vi "test4.vi"() -> ()   [LabVIEW 2014]
uses:
  <vilib>/sound2/lvsound2.llb/Sound Data Format.ctl
  <vilib>/sound2/lvsound2.llb/Sound Output Set Volume (Single).vi
  <vilib>/Utility/inputDevices.llb/keyboardAcquire.vi
  <vilib>/sound2/lvsound2.llb/Sound Output Write (DBL Single).vi
  <vilib>/Utility/inputDevices.llb/closeKeyboard.vi
  <vilib>/measure/NI_MABase.lvlib
panel:
  out "element":T1(ring)
  in  "volume":dbl=100.0
  in  "stop":bool
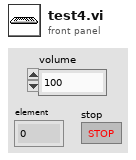
[diagram p1: front panel]
types:
  T1 = enum16{"0", "1", "2", "3", "4", "5", "6", "7", "8", "9", "A", "B", "C", "D", "E", "F", "G", "H", "I", "J", "K", "L", "M", "N", "O", "P", "Q", "R", "S", "T", "U", "V", "W", "X", "Y", "Z", "F1", "F2", "F3", "F4", "F5", "F6", "F7", "F8", "F9", "F10", "F11", "F12", "F13", "F14", "F15", "ADD", "BACK", "BACKSLASH", "CAPITAL", "COMMA", "DECIMAL", "DELETE", "DIVIDE", "DOWN", "END", "EQUALS", "ESCAPE", "GRAVE (`)", "HOME", "INSERT", "LBRACKET", "LCONTROL", "LEFT", "L ALT", "LSHIFT", "LWIN", "MINUS", "MULTIPLY", "NEXT", "NUMLOCK", "NUMPAD_0", "NUMPAD_1", "NUMPAD_2", "NUMPAD_3", "NUMPAD_4", "NUMPAD_5", "NUMPAD_6", "NUMPAD_7", "NUMPAD_8", "NUMPAD_9", "PAUSE", "PERIOD", "PRIOR (PG UP)", "RBRACKET", "RCONTROL", "RETURN", "RIGHT", "R ALT", "RSHIFT", "RWIN", "SCROLL", "SEMICOLON", "SLASH", "SPACE", "SUBTRACT", "TAB", "UP", "ENTER (num pad)", "' (quote)"}
  T2 = typedef "Sound Data Format.ctl" = cluster{"sample rate (S/s)":dbl, "number of channels":i32, "bits per sample":i32}
  T3 = typedef "Sound Output Task ID.ctl" = u32
  T4 = cluster{"sample rate (S/s)":dbl, "number of samples/ch":i32}
  T5 = enum16{"0", "1", "2", "3", "4", "5", "6", "7", "8", "9", "A", "B", "C", "D", "E", "F", "G", "H", "I", "J", "K", "L", "M", "N", "O", "P", "Q", "R", "S", "T", "U", "V", "W", "X", "Y", "Z", "F1", "F2", "F3", "F4", "F5", "F6", "F7", "F8", "F9", "F10", "F11", "F12", "F13", "F14", "F15", "ADD", "BACK", "BACKSLASH", "CAPITAL", "COMMA", "DECIMAL", "DELETE", "DIVIDE", "DOWN", "END", "EQUALS", "ESCAPE", "GRAVE (`)", "HOME", "INSERT", "LBRACKET", "LCONTROL", "LEFT", "L ALT", "LSHIFT", "LWIN", "MINUS", "MULTIPLY", "NEXT", "NUMLOCK", "NUMPAD_0", "NUMPAD_1", "NUMPAD_2", "NUMPAD_3", "NUMPAD_4", "NUMPAD_5", "NUMPAD_6", "NUMPAD_7", "NUMPAD_8", "NUMPAD_9", "PAUSE", "PERIOD", "PRIOR (PG UP)", "RBRACKET", "RCONTROL", "RETURN", "RIGHT", "R ALT", "RSHIFT", "RWIN", "SCROLL", "SEMICOLON", "SLASH", "SPACE", "SUBTRACT", "TAB", "UP", "ENTER (num pad)", "' (quote)"}[]
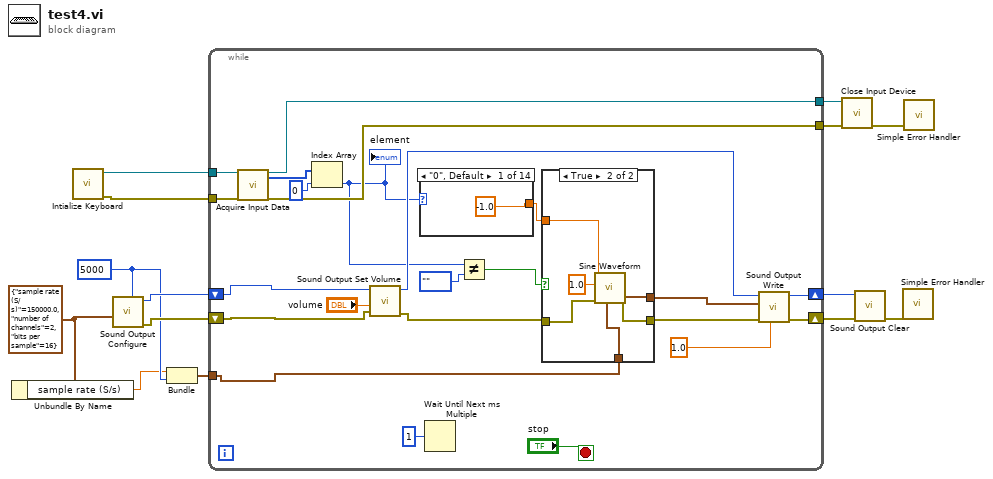
[diagram p0: block diagram]
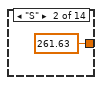
[diagram p3: hidden frame]
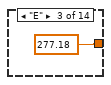
[diagram p4: hidden frame]
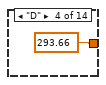
[diagram p5: hidden frame]
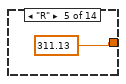
[diagram p6: hidden frame]
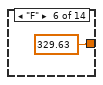
[diagram p7: hidden frame]
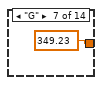
[diagram p8: hidden frame]
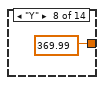
[diagram p9: hidden frame]
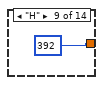
[diagram p10: hidden frame]
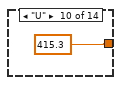
[diagram p11: hidden frame]
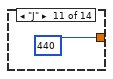
[diagram p12: hidden frame]
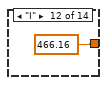
[diagram p13: hidden frame]
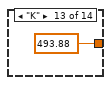
[diagram p14: hidden frame]
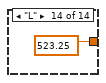
[diagram p15: hidden frame]
diagram:
  w11 = 5000 ("number of samples/ch")
  w12 = T2 {"sample rate (S/s)"=150000.0, "number of channels"=2, "bits per sample"=16} ("sound format")
  n1 = Unbundle By Name(w12) -> ("sample rate (S/s)"=w10:dbl)
  n2 = call <vilib>:"Intialize Keyboard.vi"() -> ("error out"=w4:errorcluster, "device ID"=w5:refnum<k1>)  [unwired: 10 in]
  n3 = call <vilib>:"Sound Output Configure.vi"("number of samples/ch"=w11, "sound format"=w12) -> ("error out"=w13:errorcluster, "task ID"=w14:T3)  [unwired: 8 in]
  n4 = Bundle("sample rate (S/s)"=w10, "number of samples/ch"=w11) -> (w9:T4)  [unwired: 1 in]
  n5 = while {
    tunnel: w9 -> [w26]
    shift-right: [w25] -> w8
    shift-left: w14 -> [w28]
    shift-right: [w24] -> w7
    shift-left: w13 -> [w27]
    tunnel: w5 -> [w23]
    tunnel: w4 -> [w22]
    tunnel: [w21] -> w3
    tunnel: [w20] -> w2
    stop <- "stop" stop-if-true
    n6 = call-poly <vilib>:"Acquire Input Data.vi"("device ID"=w23, "error in (no error)"=w22) -> ("device ID"=w21:refnum<k1>, "keys pressed"=w19:T5, "error out"=w20:errorcluster)  [unwired: 15 in]
    n7 = Index Array(array=w19, index=0) -> (element=w15:T1)
    "element" <- w15
    n8 = call-poly <vilib>:"Sound Output Set Volume.vi"("error in (no error)"=w27, "volume"="volume", "task ID"=w28) -> ("error out"=w30:errorcluster, "task ID out"=w29:T3)  [unwired: 7 in]
    n9 = case shown="\"0\", Default" w15 {
      tunnel: [-1.0 261.63 277.18 293.66 311.13 329.63 349.23 369.99 392 415.3 440 466.16 493.88 523.25] -> w32
      frame "0", Default {
      }
      frame "S" {
      }
      frame "E" {
      }
      frame "D" {
      }
      frame "R" {
      }
      frame "F" {
      }
      frame "G" {
      }
      frame "Y" {
      }
      frame "H" {
      }
      frame "U" {
      }
      frame "J" {
      }
      frame "I" {
      }
      frame "K" {
      }
      frame "L" {
      }
    }
    n10 = Wait Until Next ms Multiple(millisecond multiple=u32 1) -> ()  [unwired: 1 out]
    n11 = Not Equal?(x=w15, y=enum16{""}."") -> (x != y?=w16:bool)
    n12 = case shown="True" w16 {
      tunnel: w30 -> [w38 w43]
      tunnel: [_ w42] -> w35
      tunnel: [w38 w41] -> w34
      tunnel: w26 -> [_ w40]
      tunnel: w32 -> [_ w39]
      frame False {
      }
      frame True {
        n13 = call <vilib>:"Sine Waveform.vi"("sampling info"=w40, "error in (no error)"=w43, "amplitude"=1.0, "frequency"=w39) -> ("error out"=w41:errorcluster, "signal out"=w42:waveform(dbl))  [unwired: 6 in]
      }
    }
    n14 = call-poly <vilib>:"Sound Output Write.vi"("timeout (sec)"=1.0, "error in (no error)"=w34, "data"=w35, "task ID"=w29) -> ("error out"=w24:errorcluster, "task ID out"=w25:T3)  [unwired: 6 in]
  }
  n15 = call-poly <vilib>:"Close Input Device.vi"("error in (no error)"=w2, "device ID"=w3) -> ("error out"=w1:errorcluster)  [unwired: 8 in]
  n16 = call <vilib>:"Sound Output Clear.vi"("error in (no error)"=w7, "task ID"=w8) -> ("error out"=w6:errorcluster)  [unwired: 9 in]
  n17 = call <vilib>:"Simple Error Handler.vi"("error in (no error)"=w6) -> ()  [unwired: 4 in, 5 out]
  n18 = call <vilib>:"Simple Error Handler.vi"("error in (no error)"=w1) -> ()  [unwired: 4 in, 5 out]
